vi "Create_VI_Documentation_Component_Image.vi"(6 "special chars in file path of image":string, 7 "Content Options":T1, 8 "error in (no error)":errorcluster, 9 "Image Depth":i32=24, 10 "Image Format (jpeg)":enum32{"PNG", "JPEG", "GIF"}(ring)=enum."JPEG", 11 "VI":refnum<vi>) -> (0 "error out":errorcluster, 3 "Path to image":path)   [LabVIEW 2020, in "NI_ReportGenerationCore.lvlib"]
uses:
  <vilib>/Utility/NIReport.llb/NI_ReportGenerationCore.lvlib
  <vilib>/printing/ReportDocExtensions.llb/File_types_for_reports.ctl
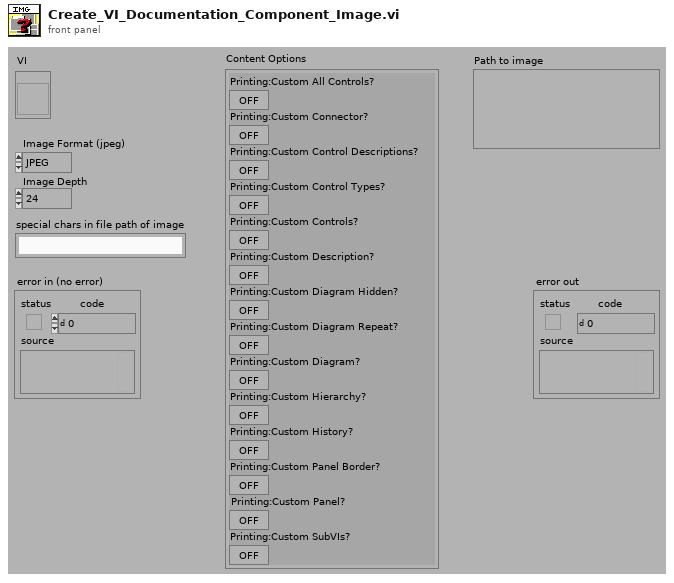
[diagram p1: front panel]
types:
  T1 = cluster{"Printing:Custom All Controls?":bool, "Printing:Custom Connector?":bool, "Printing:Custom Control Descriptions?":bool, "Printing:Custom Control Types?":bool, "Printing:Custom Controls?":bool, "Printing:Custom Description?":bool, "Printing:Custom Diagram Hidden?":bool, "Printing:Custom Diagram Repeat?":bool, "Printing:Custom Diagram?":bool, "Printing:Custom Hierarchy?":bool, "Printing:Custom History?":bool, "Printing:Custom Panel Border?":bool, "Printing:Custom Panel?":bool, "Printing:Custom SubVIs?":bool}
  T2 = typedef "NI_ReportGenerationCore.lvlib/File_types_for_reports.ctl" = enum16{".jpg", ".png", ".html", ".gif"}
  T3 = enum32{"Custom", "Standard", "Using Panel", "Using SubVI", "Complete"}
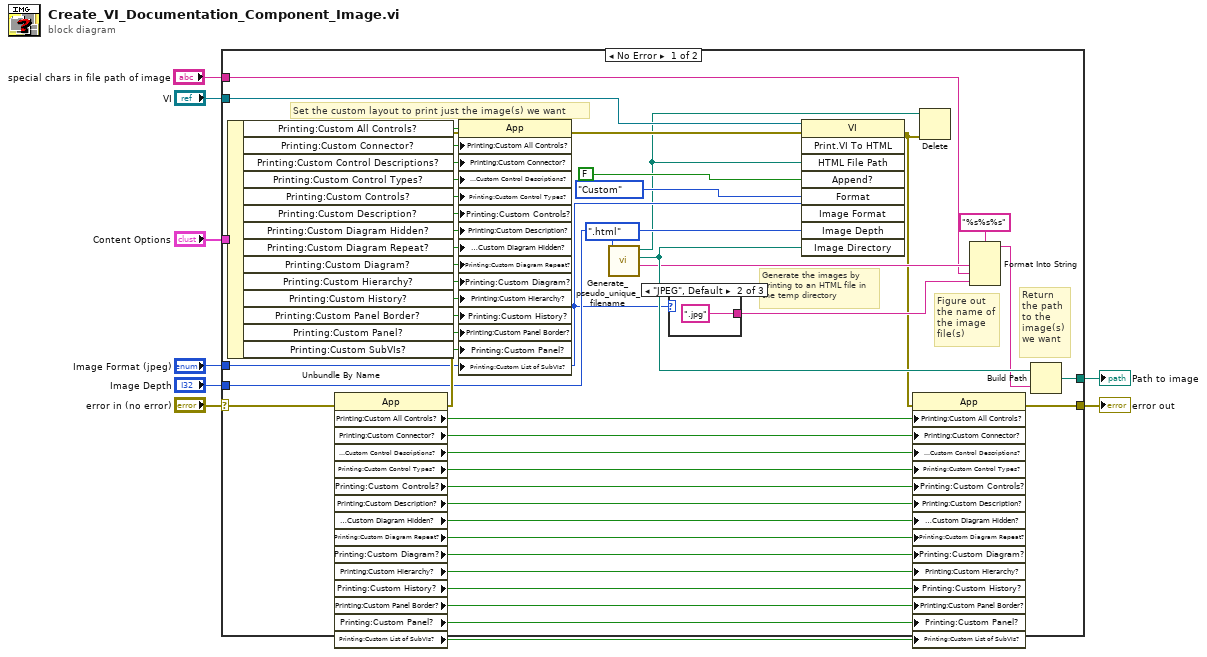
[diagram p0: block diagram]
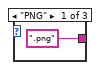
[diagram p2: hidden frame]
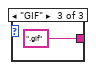
[diagram p3: hidden frame]
diagram:
  n1 = case shown="No Error" "error in (no error)" {
    selector: "error in (no error)" -> [w10 w60]
    tunnel: [w42 w60] -> w8
    tunnel: "VI" -> [w39 _]
    tunnel: "Image Depth" -> [w38 _]
    tunnel: [w31 _] -> w5
    tunnel: "Content Options" -> [w29 _]
    tunnel: "special chars in file path of image" -> [w13 _]
    tunnel: "Image Format (jpeg)" -> [w12 _]
    frame No Error {
      # "Figure out the name of the image file(s)"
      # "Return the path to the image(s) we want"
      # "Generate the images by printing to an HTML file in the temp directory"
      # "Set the custom layout to print just the image(s) we want"
      n2 = Unbundle By Name(w29) -> ("Printing:Custom All Controls?"=w28:bool, "Printing:Custom Connector?"=w27:bool, "Printing:Custom Control Descriptions?"=w26:bool, "Printing:Custom Control Types?"=w25:bool, "Printing:Custom Controls?"=w24:bool, "Printing:Custom Description?"=w23:bool, "Printing:Custom Diagram Hidden?"=w22:bool, "Printing:Custom Diagram Repeat?"=w21:bool, "Printing:Custom Diagram?"=w20:bool, "Printing:Custom Hierarchy?"=w19:bool, "Printing:Custom History?"=w18:bool, "Printing:Custom Panel Border?"=w17:bool, "Printing:Custom Panel?"=w16:bool, "Printing:Custom SubVIs?"=w15:bool)
      n3 = property class="App"(error in=w10) -> (error out=w41:errorcluster, "Printing:Custom All Controls?"=w43:bool, "Printing:Custom Connector?"=w44:bool, "Printing:Custom Control Descriptions?"=w45:bool, "Printing:Custom Control Types?"=w46:bool, "Printing:Custom Controls?"=w47:bool, "Printing:Custom Description?"=w48:bool, "Printing:Custom Diagram Hidden?"=w49:bool, "Printing:Custom Diagram Repeat?"=w50:bool, "Printing:Custom Diagram?"=w51:bool, "Printing:Custom Hierarchy?"=w52:bool, "Printing:Custom History?"=w53:bool, "Printing:Custom Panel Border?"=w54:bool, "Printing:Custom Panel?"=w55:bool, "Printing:Custom List of SubVIs?"=w56:bool)  [unwired: 1 in, 1 out]
      n4 = property class="App"(error in=w41, "Printing:Custom All Controls?"=w28, "Printing:Custom Connector?"=w27, "Printing:Custom Control Descriptions?"=w26, "Printing:Custom Control Types?"=w25, "Printing:Custom Controls?"=w24, "Printing:Custom Description?"=w23, "Printing:Custom Diagram Hidden?"=w22, "Printing:Custom Diagram Repeat?"=w21, "Printing:Custom Diagram?"=w20, "Printing:Custom Hierarchy?"=w19, "Printing:Custom History?"=w18, "Printing:Custom Panel Border?"=w17, "Printing:Custom Panel?"=w16, "Printing:Custom List of SubVIs?"=w15) -> (error out=w40:errorcluster)  [unwired: 1 in, 1 out]
      n5 = call <vilib>:"Generate_pseudo_unique_filename.vi"("file type(.jpg)"=File_types_for_reports.".html") -> ("root filename"=w30:string, "temp directory"=w33:path, "generated path"=w9:path)  [unwired: 8 in]
      n6 = case shown="\"JPEG\", Default" w12 {
        tunnel: [".png" ".jpg" ".gif"] -> w14
        frame "PNG" {
        }
        frame "JPEG", Default {
        }
        frame "GIF" {
        }
      }
      n7 = invoke class="VI" method="Print.VI To HTML"(reference=w39, error in=w40, "HTML File Path"=w9, "Append?"=FALSE, "Format"=T3."Custom", "Image Format"=w12, "Image Depth"=w38, "Image Directory"=w33) -> (error out=w11:errorcluster)  [unwired: 1 in, 8 out]
      n8 = property class="App"(error in=w11, "Printing:Custom All Controls?"=w43, "Printing:Custom Connector?"=w44, "Printing:Custom Control Descriptions?"=w45, "Printing:Custom Control Types?"=w46, "Printing:Custom Controls?"=w47, "Printing:Custom Description?"=w48, "Printing:Custom Diagram Hidden?"=w49, "Printing:Custom Diagram Repeat?"=w50, "Printing:Custom Diagram?"=w51, "Printing:Custom Hierarchy?"=w52, "Printing:Custom History?"=w53, "Printing:Custom Panel Border?"=w54, "Printing:Custom Panel?"=w55, "Printing:Custom List of SubVIs?"=w56) -> (error out=w42:errorcluster)  [unwired: 1 in, 1 out]
      n9 = Delete(path (use dialog)=w9, error in=w11) -> ()  [unwired: 3 in, 3 out]
      n10 = Format Into String(format string="%s%s%s" ("Format String"), w30, w13, w14) -> (resulting string=w32:string)  [unwired: 2 in, 1 out]
      n11 = Build Path(base path=w33, name or relative path=w32) -> (appended path=w31:path)
    }
    frame Error {
    }
  }
  "error out" <- w8
  "Path to image" <- w5
